vi "OneSensorMagazineLogic.vi"(0 "Intake Button":bool, 1 "Outtake Button":bool, 2 "Both Sensors Active":bool) -> (3 "Intake Motor":dbl, 4 "Magazine Motor":dbl, 5 "Kicker Motor":dbl, 6 "Intake Pistons":bool)   [LabVIEW 2020]
uses:
  MagazineControl New.ctl
panel:
  in  "Kicker Power":dbl=-1.0
  in  "Magazine Power":dbl=1.0
  in  "Intake Power":dbl=1.0
  # "Inputs"
  # "Power Levels"
  # "Outputs"
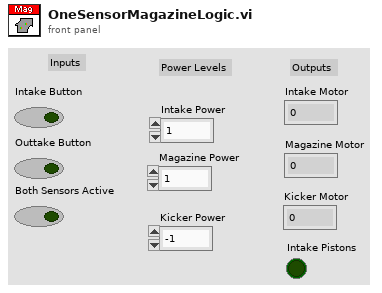
[diagram p1: front panel]
types:
  T1 = typedef "MagazineControl New.ctl" = enum16{"Idle", "Intake", "Outtake"}
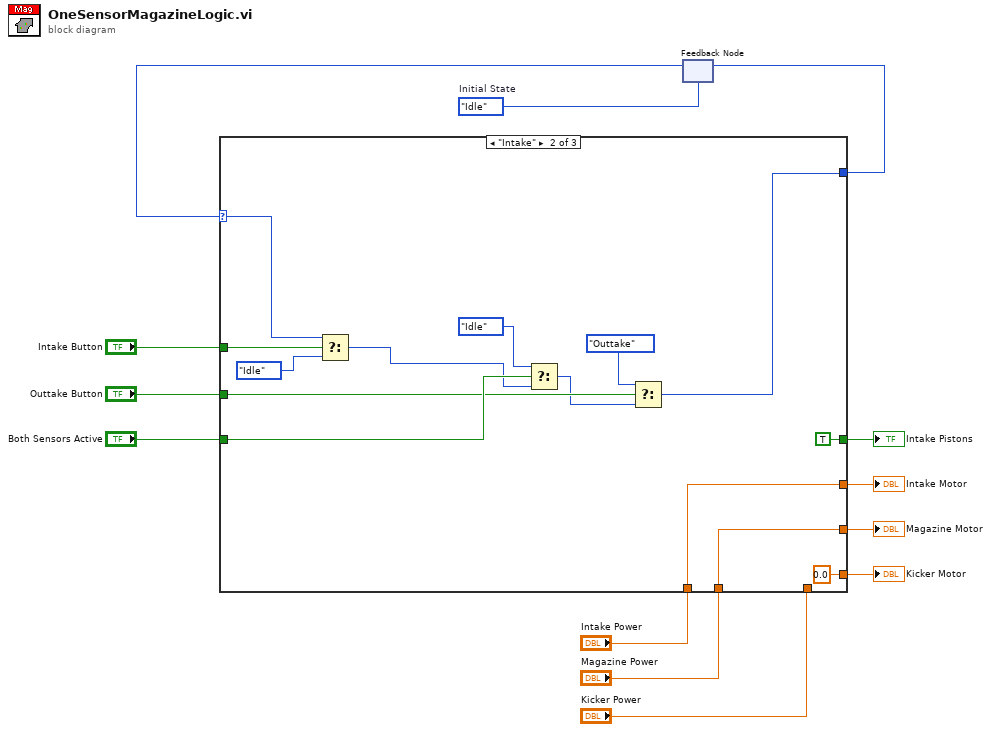
[diagram p0: block diagram]
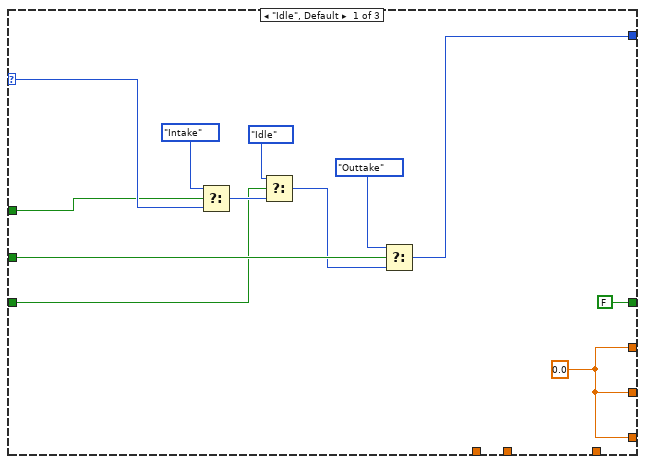
[diagram p2: hidden frame]
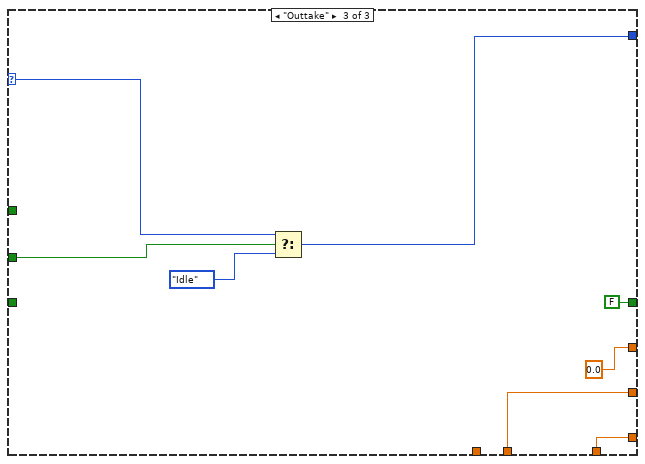
[diagram p3: hidden frame]
diagram:
  w2 = MagazineControl_New."Idle"  # Initial State
  n1 = feedback #1(w2) -> (w4:T1)
  n2 = case shown="\"Intake\"" w4 {
    selector: w4 -> [w24 w38 w40]
    tunnel: "Intake Button" -> [w18 w39 _]
    tunnel: "Outtake Button" -> [w25 w28 w47]
    tunnel: "Both Sensors Active" -> [w15 w36 _]
    tunnel: [w23 w33 0.0 ("Input Power")] -> w8
    tunnel: "Intake Power" -> [_ w33 _]
    tunnel: [w23 w32 w45] -> w10
    tunnel: "Magazine Power" -> [_ w32 w45]
    tunnel: [w23 0.0 ("Kicker Power") w42] -> w12
    tunnel: "Kicker Power" -> [_ _ w42]
    tunnel: [FALSE ("Intake Pistons") TRUE ("Intake Pistons") FALSE ("Intake Pistons")] -> w3
    tunnel: [w19 w26 w41] -> w1
    frame "Idle", Default {
      w23 = 0.0 ("Input Power")
      n3 = Select(t=MagazineControl_New."Intake", s=w18, f=w24) -> (s? t:f=w17:T1)
      n4 = Select(t=MagazineControl_New."Idle", s=w15, f=w17) -> (s? t:f=w14:T1)
      n5 = Select(t=MagazineControl_New."Outtake", s=w25, f=w14) -> (s? t:f=w19:T1)
    }
    frame "Intake" {
      n6 = Select(t=w38, s=w39, f=MagazineControl_New."Idle" ("t")) -> (s? t:f=w29:T1)
      n7 = Select(t=MagazineControl_New."Idle", s=w36, f=w29) -> (s? t:f=w27:T1)
      n8 = Select(t=MagazineControl_New."Outtake", s=w28, f=w27) -> (s? t:f=w26:T1)
    }
    frame "Outtake" {
      n9 = Select(t=w40, s=w47, f=MagazineControl_New."Idle" ("t")) -> (s? t:f=w41:T1)
    }
  }
  "Intake Motor" <- w8
  "Magazine Motor" <- w10
  "Kicker Motor" <- w12
  "Intake Pistons" <- w3
  n10 = feedback-in #1(w1) -> ()
